vi "Get Data.vi"(7 "error in (no error)":errorcluster, 10 "Device in":refnum<class "Device.lvclass">) -> (0 "error out":errorcluster, 2 "Table Indicator":string[][](table), 3 "Device out":refnum<class "Device.lvclass">)   [LabVIEW 2013, in "Device.lvclass"]
uses:
  Device.lvclass
  Device.lvclass/Device.ctl
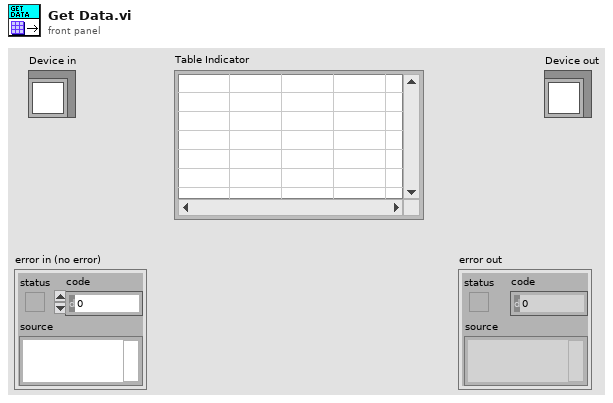
[diagram p1: front panel]
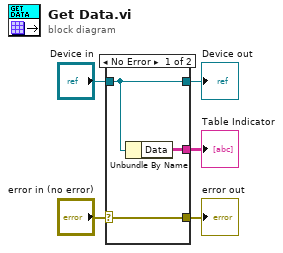
[diagram p0: block diagram]
diagram:
  n1 = case shown="No Error" "error in (no error)" {
    selector: "error in (no error)" -> [w8 w9]
    tunnel: [w8 w9] -> w4
    tunnel: "Device in" -> [w7 w10]
    tunnel: [w7 w10] -> w2
    tunnel: [w6 _] -> w1
    frame No Error {
      n2 = Unbundle By Name(w7) -> ("Data"=w6:string[][])
    }
    frame Error {
    }
  }
  "error out" <- w4
  "Table Indicator" <- w1
  "Device out" <- w2
